vi "loops.vi"() -> ()   [LabVIEW 2023]
panel:
  out "Waveform Chart 2":T1(graph)
  out "Waveform Chart":dbl[][](graph)
  in  "Numeric":i32
  out "number (0 to 1)":dbl format="%#.6g"
  in  "error in (no error)":errorcluster
  in  "y 2":bool
  in  "y":bool
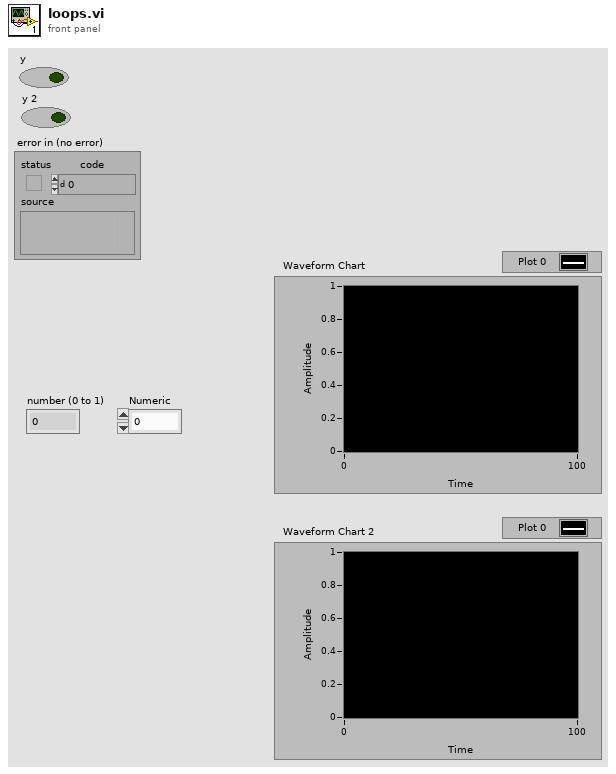
[diagram p1: front panel]
types:
  T1 = cluster{"number: 0 to 1":dbl, "number: 0 to 1":dbl}
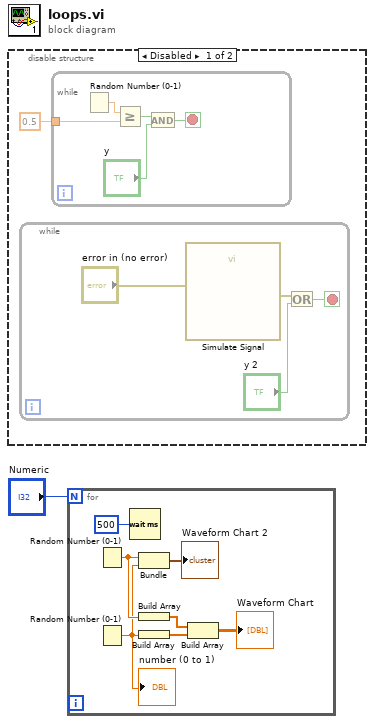
[diagram p0: block diagram]
diagram:
  n1 = disable-structure shown="Disabled" {
    frame Disabled {
      n2 = while {
        stop <- w4 stop-if-true
        n3 = call "Simulate Signal"("error in (no error)"="error in (no error)") -> ("error out"=w6:errorcluster)  [unwired: 13 in, 1 out]
        n4 = Or(x=w6, y="y 2") -> (x .or. y?=w4:bool)
      }
      n5 = while {
        tunnel: 0.5 -> [w11]
        stop <- w8 stop-if-true
        n6 = Random Number (0-1)() -> (number: 0 to 1=w7:dbl)
        n7 = Greater Or Equal?(x=w7, y=w11) -> (x >= y?=w10:bool)
        n8 = And(x=w10, y="y") -> (x .and. y?=w8:bool)
      }
    }
    frame Enabled {
    }
  }
  n9 = for {
    N: "Numeric" -> [_]
    n10 = Random Number (0-1)() -> (number: 0 to 1=w14:dbl)
    n11 = Random Number (0-1)() -> (number: 0 to 1=w13:dbl)
    "number (0 to 1)" <- w13
    n12 = Wait (ms)(milliseconds to wait=u32 500) -> ()  [unwired: 1 out]
    n13 = Bundle("number: 0 to 1"=w14, "number: 0 to 1"=w13) -> (→"Waveform Chart 2":T1)  [unwired: 1 in]
    n14 = Build Array(w14) -> (w16:dbl[])
    n15 = Build Array(w13) -> (w17:dbl[])
    n16 = Build Array(w16, w17) -> (→"Waveform Chart":dbl[][])
  }
